vi "write_gate_command.vi"() -> ()   [LabVIEW 2013]
uses:
  mcs_channel.ctl
panel:
  in  "Gate Cluster":T1 {"Threshold (V)" min=-2.5 max=2.5 step=0.001}
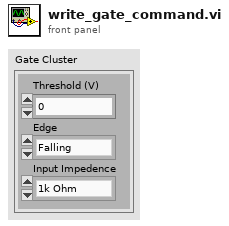
[diagram p1: front panel]
types:
  T1 = typedef "mcs_channel.ctl" = cluster{"Threshold (V)":dbl, "Edge":enum16{"Falling", "Rising"}, "Input Impedence":enum16{"1k Ohm", "50 Ohm"}}
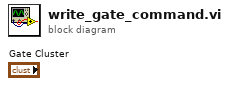
[diagram p0: block diagram]
diagram:
